vi "get handle.vi"(8 "error in (no error)":errorcluster, 11 "someclass in":refnum<class "someclass.lvclass">) -> (0 "error out":errorcluster, 2 "handle":dbl, 3 "someclass out":refnum<class "someclass.lvclass">)   [LabVIEW 2023, in "somelib.lvlib" / "someclass.lvclass"]
uses:
  someclass.lvclass
  someclass.lvclass/someclass.ctl
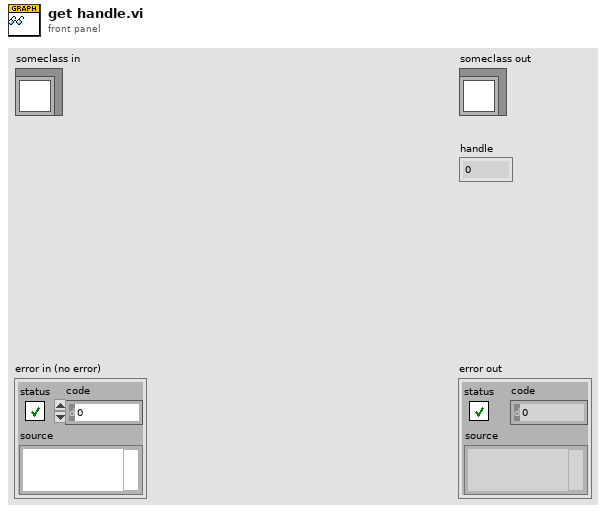
[diagram p1: front panel]
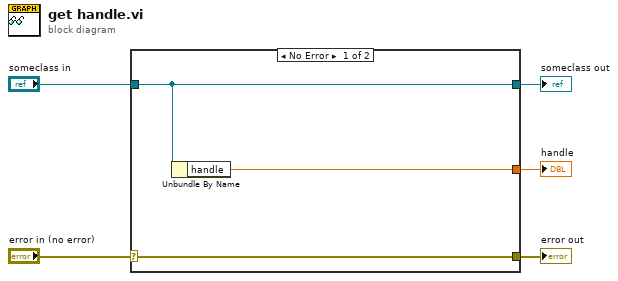
[diagram p0: block diagram]
diagram:
  n1 = case shown="No Error" "error in (no error)" {
    selector: "error in (no error)" -> [w8 w9]
    tunnel: [w8 w9] -> w4
    tunnel: [w7 w10] -> w2
    tunnel: "someclass in" -> [w7 w10]
    tunnel: [w6 _] -> w1
    frame No Error {
      n2 = Unbundle By Name(w7) -> ("handle"=w6:dbl)
    }
    frame Error {
    }
  }
  "error out" <- w4
  "someclass out" <- w2
  "handle" <- w1
